vi "Add Item.vi"(8 "error in (no error)":errorcluster, 10 "Item":refnum<class "Item.lvclass">, 11 "Listbox in":refnum<class "Listbox.lvclass">) -> (0 "error out":errorcluster, 3 "Listbox out":refnum<class "Listbox.lvclass">)   [LabVIEW 2016, in "斯坦道氨氮.lvlib" / "Listbox.lvclass"]
uses:
  Listbox.lvclass
  Interfaces/Item/Item.lvclass
  Listbox Item/Listbox Item.lvclass
  Listbox.lvclass/Listbox.ctl
  Listbox Item/Listbox Item.lvclass/Listbox Item.ctl
  <vilib>/Utility/error.llb/Error Cluster From Error Code.vi
  <vilib>/ErrorRing/Error Ring.xnode
panel:
  # "NOTICE -- YOU MUST LEAVE THIS NOTICE IN PLACE.\n\nCopyright (c) 2017, LIANG LIU Shawn.Liu.cn@gmail.com\nAll rights reserved.\n\nRedistribution and use in source and binary forms, with or without modification, are permitted provided that the following conditions are met:\n-Redistributions of source code must retain the above copyright notice, this list of conditions and the following disclaimer.\n-Redistributions in binary form must reproduce the above copyright notice, this list of conditions and the following disclaimer in the documentation and/or other materials provided with the distribution.\n-Neither the name of the eLp nor the names of its contributors may be used to endorse or promote products derived from this software without specific prior written permission.\n\nTHIS SOFTWARE IS PROVIDED BY THE COPYRIGHT HOLDERS AND CONTRIBUTORS \"AS IS\" AND ANY EXPRESS OR IMPLIED WARRANTIES, INCLUDING, BUT NOT LIMITED TO, THE IMPLIED WARRANTIES OF MERCHANTABILITY AND FITNESS FOR A PARTICULAR PURPOSE ARE DISCLAIMED. IN NO EVENT SHALL THE COPYRIGHT HOLDER OR CONTRIBUTORS BE LIABLE FOR ANY DIRECT, INDIRECT, INCIDENTAL, SPECIAL, EXEMPLARY, OR CONSEQUENTIAL DAMAGES (INCLUDING, BUT NOT LIMITED TO, PROCUREMENT OF SUBSTITUTE GOODS OR SERVICES; LOSS OF USE, DATA, OR PROFITS; OR BUSINESS INTERRUPTION) HOWEVER CAUSED AND ON ANY THEORY OF LIABILITY, WHETHER IN CONTRACT, STRICT LIABILITY, OR TORT (INCLUDING NEGLIGENCE OR OTHERWISE) ARISING IN ANY WAY OUT OF THE USE OF THIS SOFTWARE, EVEN IF ADVISED OF THE POSSIBILITY OF SUCH DAMAGE."
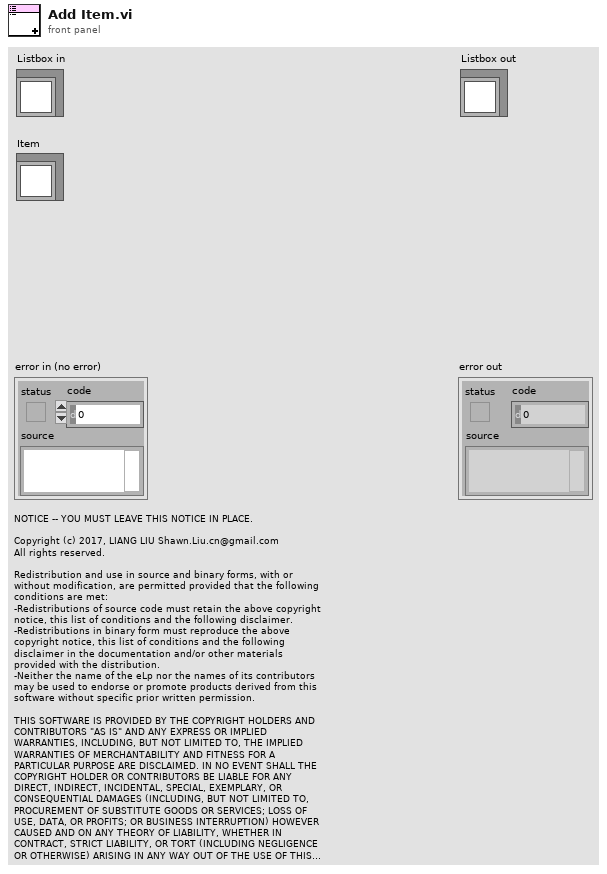
[diagram p1: front panel]
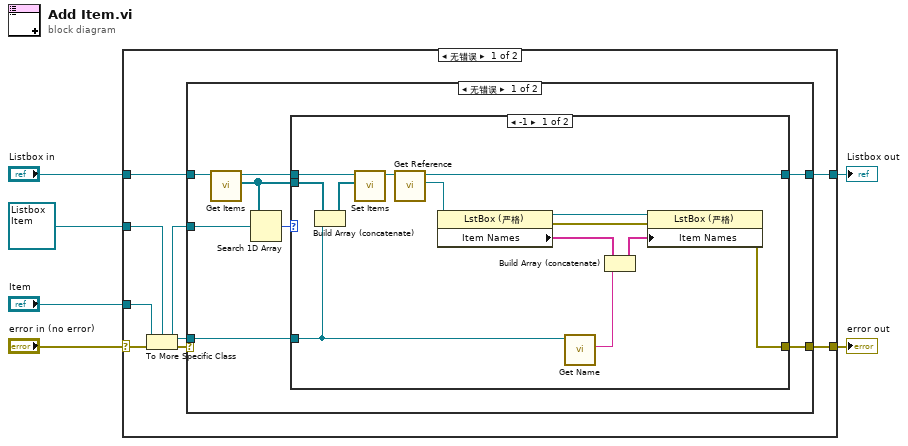
[diagram p0: block diagram]
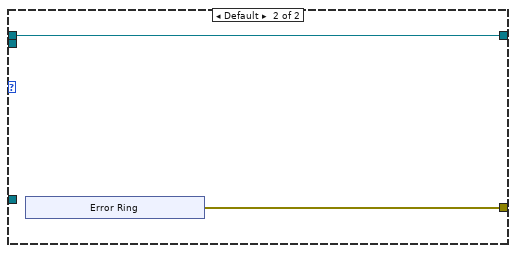
[diagram p2: hidden frame]
diagram:
  n1 = case shown="无错误" "error in (no error)" {
    selector: "error in (no error)" -> [w10 w45]
    tunnel: "Listbox in" -> [w14 w44]
    tunnel: [w13 w44] -> w5
    tunnel: refnum<class "Listbox Item.lvclass"> refnum ("Listbox Item.lvclass") -> [w12 _]
    tunnel: "Item" -> [w11 _]
    tunnel: [w9 w45] -> w1
    frame No Error {
      n2 = To More Specific Class(target class=w12, reference=w11, error in=w10) -> (specific class reference=w7:refnum<class "Listbox Item.lvclass">, error out=w8:errorcluster)
      n3 = case shown="无错误" w8 {
        selector: w8 -> [_ w43]
        tunnel: w14 -> [w22 w42]
        tunnel: [w21 w42] -> w13
        tunnel: [w20 w43] -> w9
        tunnel: w7 -> [w19 _]
        tunnel: w7 -> [w15 _]
        frame No Error {
          n4 = call "Get Items.vi"("Listbox in"=w22) -> ("Items"=w17:refnum<class "Listbox Item.lvclass">[], "Listbox out"=w18:refnum<class "Listbox.lvclass">)  [unwired: 9 in]
          n5 = Search 1D Array(1D array=w17, element=w19) -> (index of element=w16:i32)  [unwired: 1 in]
          n6 = case shown="-1" w16 {
            tunnel: [w35 w37] -> w21
            tunnel: [w34 w36] -> w20
            tunnel: w15 -> [w33 _]
            tunnel: w18 -> [w32 w37]
            tunnel: w17 -> [w31 _]
            frame -1 {
              n7 = Build Array (concatenate)(w31, w33) -> (w23:refnum<class "Listbox Item.lvclass">[])
              n8 = call "Set Items.vi"("Items"=w23, "Listbox in"=w32) -> ("Listbox out"=w24:refnum<class "Listbox.lvclass">)  [unwired: 9 in]
              n9 = call "Get Reference.vi"("Listbox in"=w24) -> ("Reference"=w29:refnum<vi>, "Listbox out"=w35:refnum<class "Listbox.lvclass">)  [unwired: 9 in]
              n10 = property class="LstBox (严格)"(reference=w29) -> (reference out=w30:refnum<vi>, error out=w28:errorcluster, "Item Names"=w27:string[])  [unwired: 1 in]
              n11 = call "Get Name.vi"("Listbox Item in"=w33) -> ("Name"=w25:string)  [unwired: 9 in, 1 out]
              n12 = Build Array (concatenate)(w27, w25) -> (w26:string[])
              n13 = property class="LstBox (严格)"(reference=w30, error in=w28, "Item Names"=w26) -> (error out=w34:errorcluster)  [unwired: 1 out]
            }
            frame Default {
              n14 = xnode "Error Ring"() -> ("错误输出"=w36:errorcluster)
            }
          }
        }
        frame Error {
        }
      }
    }
    frame Error {
    }
  }
  "error out" <- w1
  "Listbox out" <- w5
